vi "SRS-DG535_Initializer.vi"(8 "error in (no error)":errorcluster, 10 "DG535_Configs":T1 {"Trigger"."External  Level" min=-2.56 max=2.56 format="%.2f"; "Trigger"."Internal/Burst Rate" min=0.001 max=1000000.0 format="%.3f"; "Delays"."Delay" format="%#_6p"; "Output"."Offset" min=-3.0 max=4.0 format="%.2f"; "Output"."Amplitude" min=-3.0 max=4.0 format="%.2f"}, 11 "Queue in":refnum<queue>) -> (0 "error out":errorcluster, 3 "Queue out":refnum<queue>)   [LabVIEW 2013]
uses:
  <instrlib>/DG535/Command/DG535_States.ctl
  <instrlib>/DG535/DG535_Configs.ctl
  <instrlib>/DG535/Command/Set Trigger.ctl
  <instrlib>/DG535/Command/DG535_TriggerMode.ctl
  <instrlib>/DG535/Command/Set Delay.ctl
  <instrlib>/DG535/Command/DG535_Channel.ctl
  <instrlib>/DG535/Command/Set Output.ctl
  <instrlib>/DG535/Command/DG535_Output.ctl
  <instrlib>/DG535/SRS_DG535_Lib.lvlib
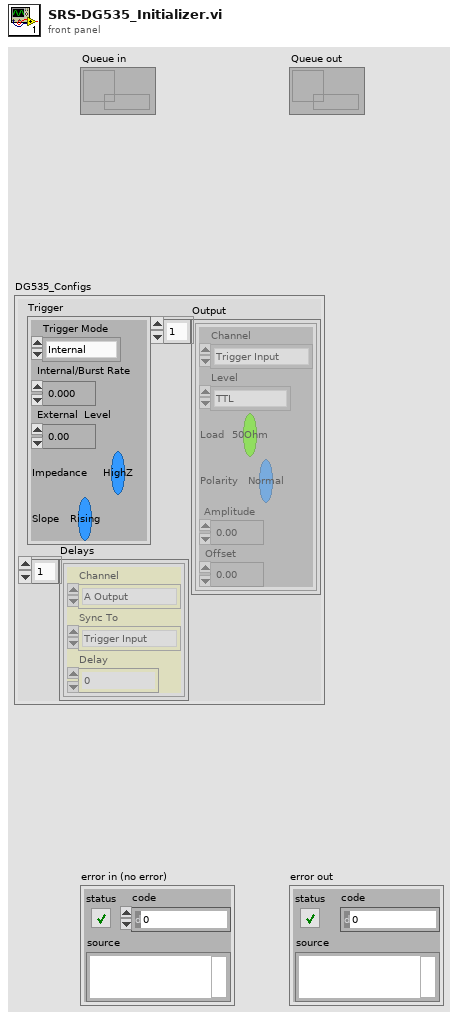
[diagram p1: front panel]
types:
  T1 = typedef "SRS_DG535_Lib.lvlib/DG535_Configs.ctl" = cluster{"Trigger":T2, "Delays":T4[], "Output":T6[]}
  T2 = typedef "SRS_DG535_Lib.lvlib/Set Trigger.ctl" = cluster{"Trigger Mode":T3, "Internal/Burst Rate":dbl, "External  Level":sgl, "Impedance":bool, "Slope":bool}
  T3 = typedef "SRS_DG535_Lib.lvlib/DG535_TriggerMode.ctl" = enum16{"Internal", "External", "SingleShot", "Burst", "Line"}
  T4 = typedef "SRS_DG535_Lib.lvlib/Set Delay.ctl" = cluster{"Channel":T5, "Sync To":T5, "Delay":dbl}
  T5 = typedef "SRS_DG535_Lib.lvlib/DG535_Channel.ctl" = enum16{"Trigger Input", "T0 Output", "A Output", "B Output", "AB Output", "C Output", "D Output", "CD Output", "NULL"}
  T6 = typedef "SRS_DG535_Lib.lvlib/Set Output.ctl" = cluster{"Channel":T5, "Level":T7, "Load":bool, "Polarity":bool, "Amplitude":dbl, "Offset":dbl}
  T7 = typedef "SRS_DG535_Lib.lvlib/DG535_Output.ctl" = enum16{"TTL", "NIM", "ECL", "Variable"}
  T8 = typedef "SRS_DG535_Lib.lvlib/DG535_States.ctl" = cluster{"State":enum16{"Initialize", "Set Trigger", "Set Output", "Set Delay", "Manl_Trig", "Run", "Stop", "Close", "Quit"}, "Para.":variant}
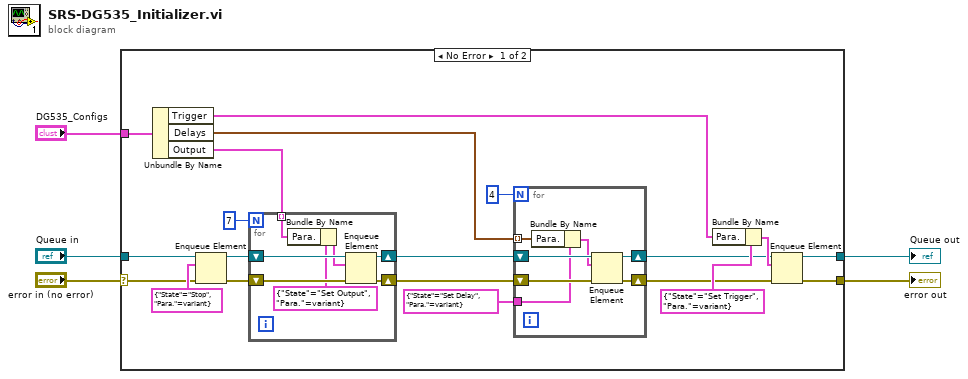
[diagram p0: block diagram]
diagram:
  n1 = case shown="No Error" "error in (no error)" {
    selector: "error in (no error)" -> [w6 w41]
    tunnel: "Queue in" -> [w25 w40]
    tunnel: "DG535_Configs" -> [w24 _]
    tunnel: [w23 w41] -> w3
    tunnel: [w22 w40] -> w2
    frame No Error {
      n2 = Unbundle By Name(w24) -> ("Trigger"=w19:T2, "Delays"=w14:T4[], "Output"=w20:T6[])
      n3 = Enqueue Element(queue=w25, element=T8 {"State"=enum."Stop", "Para."=variant}, error in (no error)=w6) -> (queue out=w7:refnum<queue>, error out=w10:errorcluster)  [unwired: 1 in, 1 out]
      n4 = for {
        N: 7 -> [_]
        shift-right: [w31] -> w8
        shift-left: w7 -> [w32]
        shift-right: [w29] -> w11
        shift-left: w10 -> [w30]
        tunnel: w20 -> [w26] mode=indexing
        n5 = Bundle By Name(cluster=T8 {"State"=enum."Set Output", "Para."=variant} ("element"), "Para."=w26) -> (w27:T8)
        n6 = Enqueue Element(queue=w32, element=w27, error in (no error)=w30) -> (queue out=w31:refnum<queue>, error out=w29:errorcluster)  [unwired: 1 in, 1 out]
      }
      n7 = for {
        N: 4 -> [_]
        shift-right: [w37] -> w16
        shift-left: w11 -> [w38]
        tunnel: T8 {"State"=enum."Set Delay", "Para."=variant} ("element") -> [w36]
        tunnel: w14 -> [w34] mode=indexing
        shift-right: [w33] -> w15
        shift-left: w8 -> [w39]
        n8 = Bundle By Name(cluster=w36, "Para."=w34) -> (w35:T8)
        n9 = Enqueue Element(queue=w39, element=w35, error in (no error)=w38) -> (queue out=w33:refnum<queue>, error out=w37:errorcluster)  [unwired: 1 in, 1 out]
      }
      n10 = Bundle By Name(cluster=T8 {"State"=enum."Set Trigger", "Para."=variant} ("element"), "Para."=w19) -> (w18:T8)
      n11 = Enqueue Element(queue=w15, element=w18, error in (no error)=w16) -> (queue out=w22:refnum<queue>, error out=w23:errorcluster)  [unwired: 1 in, 1 out]
    }
    frame Error {
    }
  }
  "error out" <- w3
  "Queue out" <- w2
